vi "Parameters from Front Panel.vi"(8 "error in (no error)":errorcluster, 11 "Mag Lab Measure Interface in":refnum<class "Mag Lab Measure UI.lvclass">) -> (0 "error out":errorcluster, 3 "Mag Lab Measure Interface out":refnum<class "Mag Lab Measure UI.lvclass">)   [LabVIEW 2015, in "Mag Lab Measure UI.lvclass"]
uses:
  Mag Lab Measure UI.lvclass
  Mag Lab Measure UI.lvclass/Mag Lab Measure UI.ctl
  Mag Lab Properties/Mag Lab Parameters.lvclass
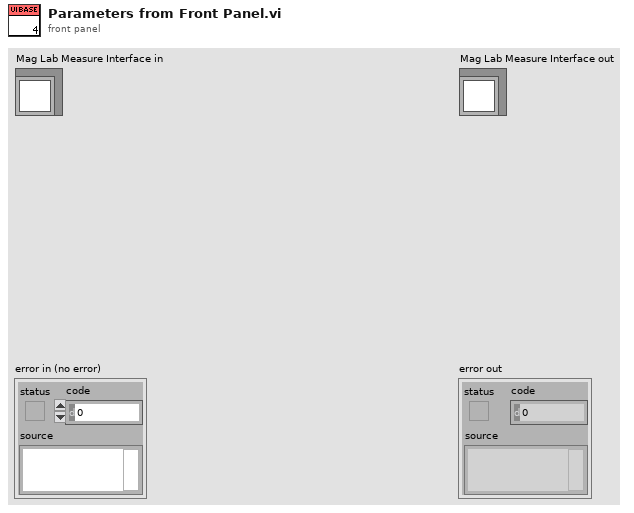
[diagram p1: front panel]
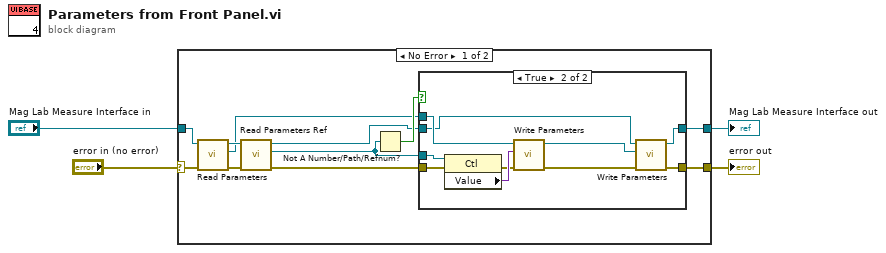
[diagram p0: block diagram]
diagram:
  n1 = case shown="No Error" "error in (no error)" {
    selector: "error in (no error)" -> [w5 w29]
    tunnel: [w13 w29] -> w3
    tunnel: [w9 w28] -> w1
    tunnel: "Mag Lab Measure Interface in" -> [w15 w28]
    frame No Error {
      n2 = call-dynamic "Read Parameters.vi"("error in (no error)"=w5, "Mag Lab Root in"=w15) -> ("error out"=w6:errorcluster, "Mag Lab Parameters.lvclass"=w7:refnum<class "Mag Lab Parameters.lvclass">, "Mag Lab Root out"=w8:refnum<class "Mag Lab Measure UI.lvclass">)  [unwired: 7 in]
      n3 = call "Read Parameters Ref.vi"("error in (no error)"=w6, "Mag Lab Measure Interface in"=w8) -> ("error out"=w14:errorcluster, "Parameters"=w12:refnum<vi>, "Mag Lab Measure Interface out"=w10:refnum<class "Mag Lab Measure UI.lvclass">)  [unwired: 7 in]
      n4 = Not A Number/Path/Refnum?(number/path/refnum=w12) -> (NaN/Path/Refnum?=w11:bool)
      n5 = case shown="True" w11 {
        tunnel: w12 -> [_ w27]
        tunnel: w14 -> [w17 w26]
        tunnel: [w17 w18] -> w13
        tunnel: w7 -> [_ w23]
        tunnel: w10 -> [w16 w20]
        tunnel: [w16 w19] -> w9
        frame False {
        }
        frame True {
          n6 = property class="Ctl"(reference=w27, error in=w26) -> (error out=w24:errorcluster, "Value"=w25:variant)  [unwired: 1 out]
          n7 = call-dynamic "Write Parameters.vi"("error in (no error)"=w24, "Parameters"=w25, "Mag Lab Parameters in"=w23) -> ("error out"=w22:errorcluster, "Mag Lab Parameters out"=w21:refnum<class "Mag Lab Parameters.lvclass">)  [unwired: 7 in]
          n8 = call-dynamic "Write Parameters.vi"("error in (no error)"=w22, "Mag Lab Parameters.lvclass"=w21, "Mag Lab Root in"=w20) -> ("error out"=w18:errorcluster, "Mag Lab Root out"=w19:refnum<class "Mag Lab Measure UI.lvclass">)  [unwired: 7 in]
        }
      }
    }
    frame Error {
    }
  }
  "error out" <- w3
  "Mag Lab Measure Interface out" <- w1
